vi "Graphics-Rotate Pixmap and Mask.vi"(8 "Angle (degrees)":dbl, 10 "mask":bool[][](array[boolean]), 11 "24-bit pixmap":u32[][](array[numeric])) -> (2 "rotated mask":u8[](array[numeric]), 3 "rotated pixmap":u32[][](array[numeric]))   [LabVIEW 2015]
uses:
  PXI DAQ VIs/Utility VIs/Array Dimensions (2D).vi
panel:
  out "size(s)":i32
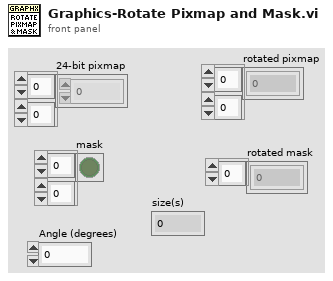
[diagram p1: front panel]
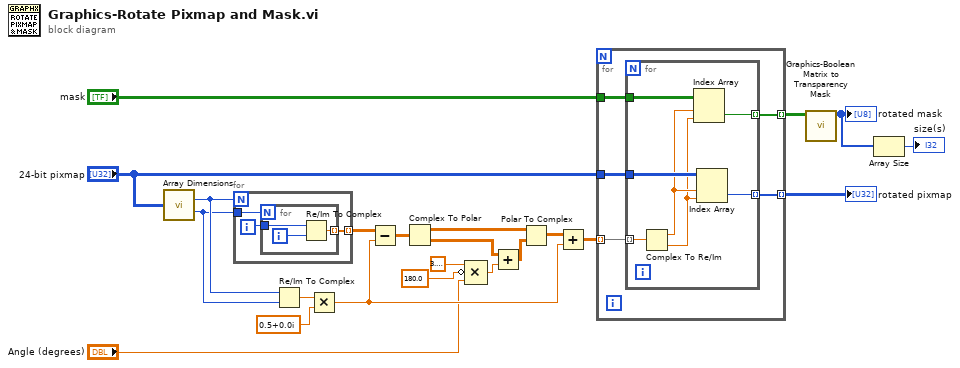
[diagram p0: block diagram]
diagram:
  n1 = call-poly "Array Dimensions.vi"("2D Array"="24-bit pixmap") -> ("# rows"=w8:i32, "# columns"=w7:i32)  [unwired: 13 in]
  n2 = for {
    N: w8 -> [_]
    tunnel: w7 -> [w25]
    tunnel: [w23] -> w18 mode=indexing
    i -> [w24]
    n3 = for {
      N: w25 -> [_]
      tunnel: w24 -> [w27]
      tunnel: [w26] -> w23 mode=indexing
      i -> [w28]
      n4 = Re/Im To Complex(1:w28, 2:w27) -> (0:w26:cdb)
    }
  }
  n5 = Re/Im To Complex(1:w7, 2:w8) -> (0:w16:cdb)
  n6 = Multiply(x=w16, y=cdb 0.5+0.0i) -> (x*y=w22:cdb)
  n7 = Subtract(x=w18, y=w22) -> (x-y=w19:cdb[][])
  n8 = Complex To Polar(r * e^(i*theta)=w19) -> (r=w20:dbl[][], theta=w21:dbl[][])
  n9 = Compound Arithmetic op=MULTIPLY(3.141592653589793, invert 180.0, "Angle (degrees)") -> (w13:dbl)
  n10 = Add(x=w21, y=w13) -> (x+y=w12:dbl[][])
  n11 = Polar To Complex(1:w12, 2:w20) -> (0:w11:cdb[][])
  n12 = Add(x=w11, y=w22) -> (x+y=w10:cdb[][])
  n13 = for {
    tunnel: w10 -> [w33] mode=indexing
    tunnel: [w32] -> w6 mode=indexing
    tunnel: "24-bit pixmap" -> [w31]
    tunnel: "mask" -> [w30]
    tunnel: [w29] -> w4 mode=indexing
    n14 = for {
      tunnel: w33 -> [w40] mode=indexing
      tunnel: [w39] -> w32 mode=indexing
      tunnel: w31 -> [w38]
      tunnel: w30 -> [w37]
      tunnel: [w34] -> w29 mode=indexing
      n15 = Complex To Re/Im(x + iy=w40) -> (x=w36:dbl, y=w35:dbl)
      n16 = Index Array(array=w37, index (row)=w36, index (col)=w35) -> (element=w34:bool)
      n17 = Index Array(array=w38, index (row)=w36, index (col)=w35) -> (element=w39:u32)
    }
  }
  "rotated pixmap" <- w6
  n18 = call "Graphics-Boolean Matrix to Transparency Mask.vi"("Mask In"=w4) -> ("Mask Out"=w3:u8[])  [unwired: 10 in]
  "rotated mask" <- w3
  n19 = Array Size(array=w3) -> (size(s)=→"size(s)":i32)
